vi "PSU Ramp field.vi"(8 "Ramp to set [A/s]":dbl, 9 "Field to set [T]":dbl, 10 "PSU Status In":T1 {"Trip Current" format="%.3f"; "Trip Field" format="%.4f"; "Voltage" format="%.2f"; "Field Constant" format="%.6f"; "MID Setpoint (T)" format="%.4f"; "MID Setpoint (A)" format="%.3f"; "MAX Setpoint (T)" format="%.4f"; "MAX Setpoint (A)" format="%.3f"; "Heater Voltage" format="%.2f"; "V Limit (V)" format="%.2f"; "Ramp Rate (A/s)" format="%.3f"; "Output (A)" format="%.3f"; "Output (T)" format="%.4f"; "Persistent Current" format="%.3f"; "Persistent Field" format="%.4f"}, 11 "VISA Refnum in":refnum<visa-resource-name>) -> (0 "error out":errorcluster, 1 "Desired field (T)":dbl, 2 "Ramp Rate (T/s)":dbl, 3 "PSU Status Out":T1 {"Trip Current" format="%.3f"; "Trip Field" format="%.4f"; "Voltage" format="%.2f"; "Field Constant" format="%.6f"; "MID Setpoint (T)" format="%.4f"; "MID Setpoint (A)" format="%.3f"; "MAX Setpoint (T)" format="%.4f"; "MAX Setpoint (A)" format="%.3f"; "Heater Voltage" format="%.2f"; "V Limit (V)" format="%.2f"; "Ramp Rate (A/s)" format="%.3f"; "Output (A)" format="%.3f"; "Output (T)" format="%.4f"; "Persistent Current" format="%.3f"; "Persistent Field" format="%.4f"})   [LabVIEW 2017, in "Magnet module.lvlib"]
doc: "Set requeiered field and ramp. Then starts ramping.\nReturns status, destination field and ramp rate in T/s."
uses:
  Magnet module.lvlib
  <instrlib>/SMS drivers/Source Code/Public/PSU Status.ctl
  <instrlib>/SMS drivers/Source Code/Cryogenic Ltd SMSXXX.lvlib
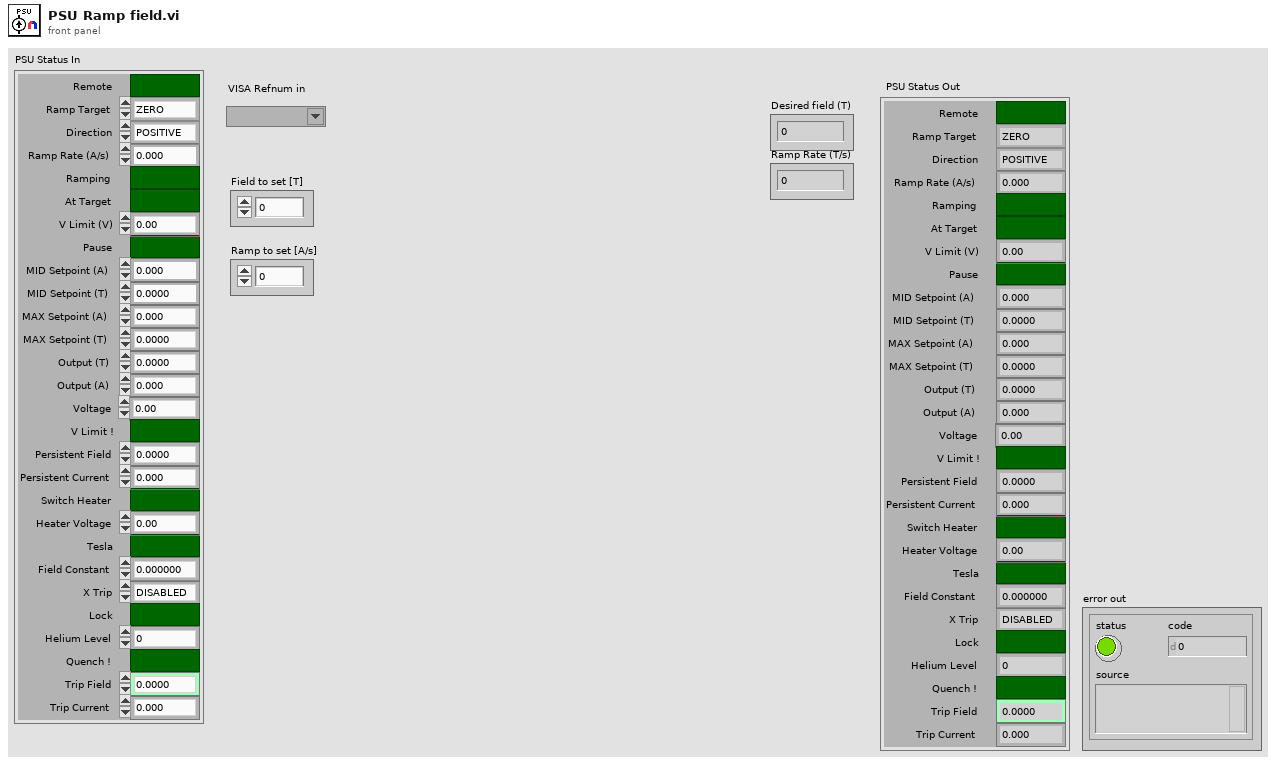
[diagram p1: front panel]
types:
  T1 = typedef "Cryogenic Ltd SMSXXX.lvlib/PSU Status.ctl" = cluster{"Ramp Target":enum16{"ZERO", "MID", "MAX"}, "Pause":bool, "Switch Heater":bool, "Persistent Field":dbl, "Persistent Current":dbl, "Tesla":bool, "Output (T)":dbl, "Output (A)":dbl, "X Trip":enum16{"DISABLED", "ENABLED", "ACTIVE"}, "Ramp Rate (A/s)":dbl, "V Limit (V)":dbl, "Heater Voltage":dbl, "MAX Setpoint (A)":dbl, "MAX Setpoint (T)":dbl, "MID Setpoint (A)":dbl, "MID Setpoint (T)":dbl, "Lock":bool, "Field Constant":dbl, "Remote":bool, "Direction":enum16{"POSITIVE", "NEGATIVE", "OPEN", "UNIPOLAR"}, "Helium Level":u16, "Quench !":bool, "Voltage":dbl, "V Limit !":bool, "Ramping":bool, "At Target":bool, "Trip Field":dbl, "Trip Current":dbl}
  T2 = enum16{"RAMP TO ZERO", "RAMP TO MID", "RAMP TO MAX"}
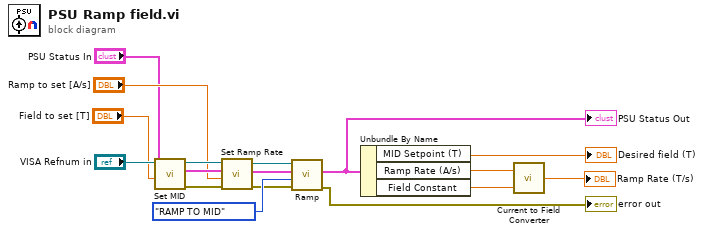
[diagram p0: block diagram]
diagram:
  n1 = call <instrlib>:"Set MID.vi"("MID (T or A)"="Field to set [T]", "PSU Status In"="PSU Status In", "VISA Resource Name In"="VISA Refnum in") -> ("Error out"=w13:errorcluster, "PSU Status Out"=w14:T1, "VISA Resource Name Out"=w9:refnum<visa-resource-name>)  [unwired: 5 in, 1 out]
  n2 = call <instrlib>:"Set Ramp Rate.vi"("Error in (no error)"=w13, "Ramp Rate (A/s)"="Ramp to set [A/s]", "PSU Status In"=w14, "VISA Resource Name In"=w9) -> ("Error out"=w12:errorcluster, "PSU Status Out"=w1:T1, "VISA Resource Name Out"=w10:refnum<visa-resource-name>)  [unwired: 4 in, 1 out]
  n3 = call <instrlib>:"Ramp.vi"("Error in (no error)"=w12, "Ramp Target"=T2."RAMP TO MID", "PSU Status In"=w1, "VISA Resource Name In"=w10) -> ("Error out"=→"error out":errorcluster, "PSU Status Out"=w7:T1)  [unwired: 4 in, 2 out]
  "PSU Status Out" <- w7
  n4 = Unbundle By Name(w7) -> ("MID Setpoint (T)"=→"Desired field (T)":dbl, "Ramp Rate (A/s)"=w4:dbl, "Field Constant"=w5:dbl)
  n5 = call "Current to Field Converter.vi"("Field constant [T/A]"=w5, "Current in [A]"=w4) -> ("Field out [T]"=→"Ramp Rate (T/s)":dbl)
